vi "DFD NStage MRate Filtering with State.vi"   [LabVIEW 2017, in "NI_DigFilterLicensed.lvlib"]
doc: "Filters a signal with a multistage multirate filter. You must specify the initial internal states in <B>state in</B> to filter the samples accurately. Wire data to the <B>signal in</B> input to determine the polymorphic instance to use or manually select the instance."
uses:
  <vilib>/addons/Digital Filter Design/NI_DigFilterLicensed.lvlib
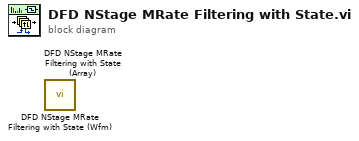
[diagram p0: block diagram]
diagram:
  n1 = call <vilib>:"DFD NStage MRate Filtering with State (Wfm).vi"() -> ()  [unwired: 9 in, 3 out]
  n2 = call <vilib>:"DFD NStage MRate Filtering with State (Array).vi"() -> ()  [unwired: 9 in, 3 out]
